vi "Cond Timed Wait (relative seconds).vi"(8 "error in (no error)":errorcluster, 9 "relative timeout (seconds)":dbl, 10 "Mutex in":T1, 11 "Cond in":T2) -> (0 "error out":errorcluster, 1 "timed out?":bool, 2 "Mutex out":T1, 3 "Cond out":T2)   [LabVIEW 2013, in "POSIX Threads.lvlib" / "Cond.lvclass"]
doc: "Calls pthread_cond_timedwait() on the pthread cond object encapsulated by Cond.\n\nThe relative timeout provided will be used to generate an absolute timeout internally before calling pthread_cond_timedwait().\n\nRefer to online POSIX documentation for more information."
uses:
  Cond.lvclass
  Controls/reference.ctl
  Mutex/Controls/reference.ctl
  Mutex/Mutex.lvclass
  Cond.lvclass/Cond.ctl
  POSIX Thread Object/POSIX Thread Object.lvclass/POSIX Thread Object.ctl
  POSIX Thread Object/Private VIs/libpthread path.vi
  <vilib>/NI/NI Linux RT Utilities/VIs/Public/Convert Types/convert timespec 64 to timespec 32.vi
  <vilib>/NI/NI Linux RT Utilities/VIs/Public/Time/Increment Time (timespec).vi
  <vilib>/NI/NI Linux RT Utilities/VIs/Public/Time/Get Clock Time (timespec).vi
  POSIX Thread Object/Private VIs/get pthread error.vi
  POSIX Thread Object/POSIX Thread Object.lvclass
  <vilib>/NI/NI Linux RT Utilities/Linux RT Utilities.lvlib
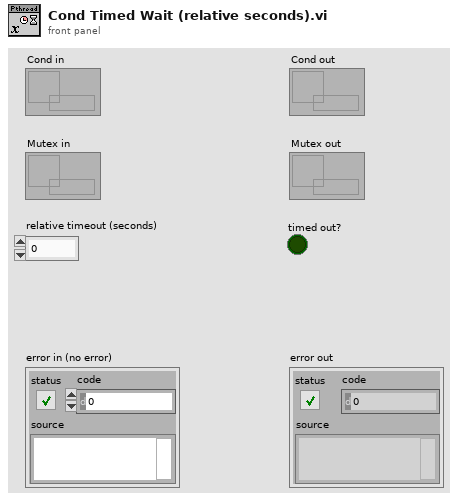
[diagram p1: front panel]
types:
  T1 = typedef "POSIX Threads.lvlib/Mutex.lvclass/reference.ctl" = refnum<data-value>
  T2 = typedef "POSIX Threads.lvlib/Cond.lvclass/reference.ctl" = refnum<data-value>
  T3 = typedef "Linux RT Utilities.lvlib/clockid_t.ctl" = enum16{"Realtime", "Monotonic"}
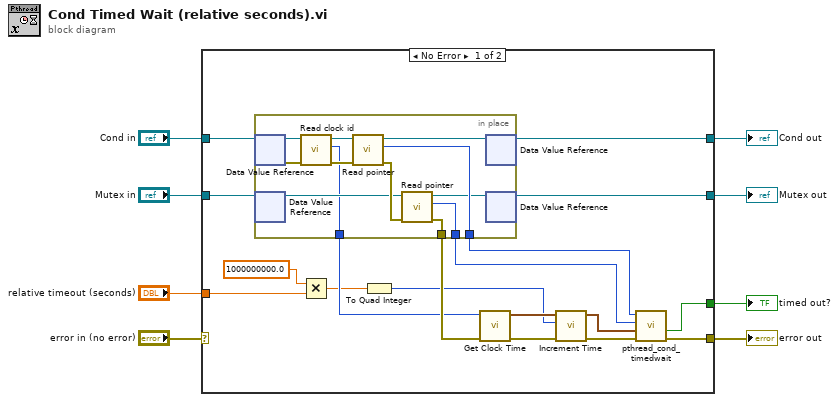
[diagram p0: block diagram]
diagram:
  n1 = case shown="No Error" "error in (no error)" {
    selector: "error in (no error)" -> [_ w41]
    tunnel: [w26 w41] -> w7
    tunnel: "Cond in" -> [w24 w40]
    tunnel: [w21 w40] -> w5
    tunnel: "Mutex in" -> [w23 w39]
    tunnel: [w20 w39] -> w3
    tunnel: "relative timeout (seconds)" -> [w11 _]
    tunnel: [w25 _] -> w1
    frame No Error {
      n2 = in-place {
        in-place-border: [w37] -> w19
        in-place-border: [w35] -> w15
        in-place-border: [w34] -> w22
        in-place-border: [w27] -> w14
        n3 = in-place-dvr #1(w24) -> (w33:refnum<class "Cond.lvclass">, w32:errorcluster)
        n4 = in-place-dvr #2(w23) -> (w28:refnum<class "Mutex.lvclass">)  [unwired: 1 out]
        n5 = call "Read clock id.vi"("error in (no error)"=w32, "Cond in"=w33) -> ("error out"=w31:errorcluster, "lv_clockid_t"=w27:T3, "Cond out"=w30:refnum<class "Cond.lvclass">)  [unwired: 7 in]
        n6 = call "Read pointer.vi"("error in (no error)"=w31, "POSIX Thread Object in"=w30) -> ("error out"=w29:errorcluster, "pointer"=w37:u64, "POSIX Thread Object out"=w38:refnum<class "Cond.lvclass">)  [unwired: 7 in]
        n7 = call "Read pointer.vi"("error in (no error)"=w29, "POSIX Thread Object in"=w28) -> ("error out"=w35:errorcluster, "pointer"=w34:u64, "POSIX Thread Object out"=w36:refnum<class "Mutex.lvclass">)  [unwired: 7 in]
        n8 = in-place-dvr #1(w38) -> (w21:T2)  [unwired: 1 out]
        n9 = in-place-dvr #2(w36) -> (w20:T1)  [unwired: 1 out]
      }
      n10 = Multiply(x=1000000000.0, y=w11) -> (x*y=w10:dbl)
      n11 = To Quad Integer(1:w10) -> (0:w9:i64)
      n12 = call-poly <vilib>:"Get Clock Time.vi"("error in (no error)"=w15, "clock id (realtime)"=w14) -> ("error out"=w17:errorcluster, "timespec"=w13:cluster{"sec":u64, "nsec":u64})  [unwired: 8 in]
      n13 = call-poly <vilib>:"Increment Time.vi"("error in (no error)"=w17, "nanoseconds to add"=w9, "timespec in"=w13) -> ("error out"=w18:errorcluster, "timespec out"=w16:cluster{"sec":u64, "nsec":u64})  [unwired: 7 in]
      n14 = call "pthread_cond_timedwait.vi"("error in (no error)"=w18, "absolute time"=w16, "mutex ptr in"=w22, "cond ptr in"=w19) -> ("error out"=w26:errorcluster, "timed out?"=w25:bool)  [unwired: 4 in, 2 out]
    }
    frame Error {
    }
  }
  "Cond out" <- w5
  "error out" <- w7
  "Mutex out" <- w3
  "timed out?" <- w1
